vi "close device.vi"(8 "error in (no error)":errorcluster, 11 "id":i32) -> (0 "error out":errorcluster, 2 "function return":i32, 3 "id out":i32)   [LabVIEW 2020, in "libximc.lvlib"]
doc: "result_t XIMC_API close_device (device_t* id);"
uses:
  libximc.lvlib
  libximc.dll
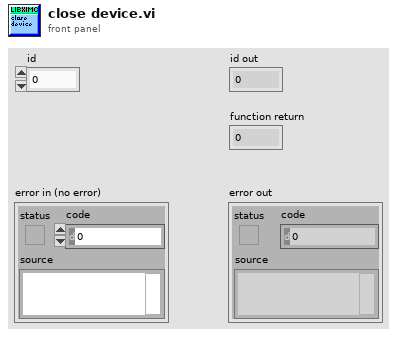
[diagram p1: front panel]
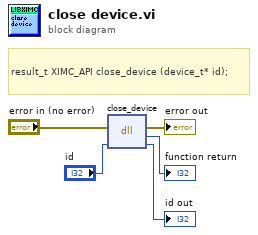
[diagram p0: block diagram]
diagram:
  # "result_t XIMC_API close_device (device_t* id);"
  n1 = dll-call lib="E:/Norway Project/All Hardware/New Microscope/LabVIEW/Stage/libximc.*" fn="close_device"(error in="error in (no error)", "id"="id") -> (error out=→"error out":errorcluster, →"function return":i32, "id"=→"id out":i32)  [unwired: 2 in, 1 out]
